vi "openCANCoders.vi"(11 "error in":errorcluster) -> (3 "output cluster":T2)   [LabVIEW 2020]
uses:
  <vilib>/Rock Robotics/WPI/ThirdParty/Phoenix-LabVIEW/CANCoder/Controls/CTRE_Phoenix_CANcoder_DeviceRef.ctl
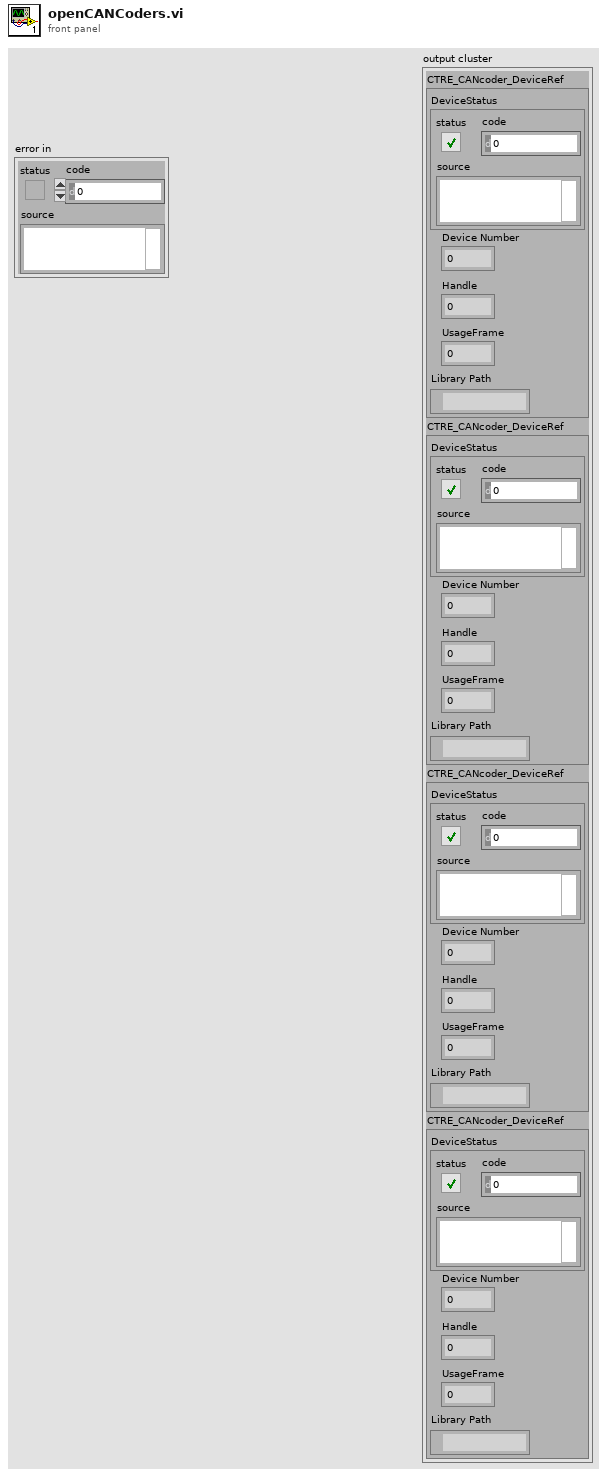
[diagram p1: front panel]
types:
  T1 = typedef "CTRE_Phoenix_CANcoder_DeviceRef.ctl" = cluster{"DeviceStatus":errorcluster, "Device Number":u8, "Handle":u64, "UsageFrame":u32, "Library Path":path}
  T2 = cluster{"CTRE_CANcoder_DeviceRef":T1, "CTRE_CANcoder_DeviceRef":T1, "CTRE_CANcoder_DeviceRef":T1, "CTRE_CANcoder_DeviceRef":T1}
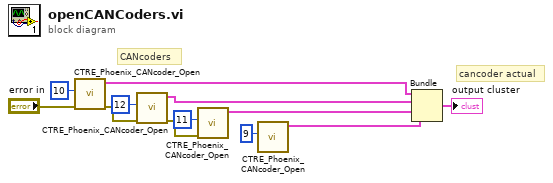
[diagram p0: block diagram]
diagram:
  # "CANcoders"
  # "cancoder actual"
  n1 = call <vilib>:"CTRE_Phoenix_CANcoder_Open.vi"("error in"="error in", "Device Number"=u8 10) -> ("error out"=w8:errorcluster, "CTRE_CANcoder_DeviceRef"=w6:T1)  [unwired: 8 in]
  n2 = call <vilib>:"CTRE_Phoenix_CANcoder_Open.vi"("error in"=w8, "Device Number"=u8 12) -> ("error out"=w7:errorcluster, "CTRE_CANcoder_DeviceRef"=w5:T1)  [unwired: 8 in]
  n3 = call <vilib>:"CTRE_Phoenix_CANcoder_Open.vi"("error in"=w7, "Device Number"=u8 11) -> ("CTRE_CANcoder_DeviceRef"=w4:T1)  [unwired: 8 in, 1 out]
  n4 = call <vilib>:"CTRE_Phoenix_CANcoder_Open.vi"("Device Number"=u8 9) -> ("CTRE_CANcoder_DeviceRef"=w3:T1)  [unwired: 9 in, 1 out]
  n5 = Bundle("CTRE_CANcoder_DeviceRef"=w6, "CTRE_CANcoder_DeviceRef"=w5, "CTRE_CANcoder_DeviceRef"=w4, "CTRE_CANcoder_DeviceRef"=w3) -> (→"output cluster":T2)  [unwired: 1 in]
